vi "XY Plot Commands.vi"(1 "X,Y Log":i32[](array[numeric])=[1, 0], 4 "Plot labels":string[](array[string])=["SR810 cables", "SR810 cables + 1&2", "detector", "cables", "cables + 1&2", "cables + 2&3", "cables + 3&4"], 5 "X,Y Labels":string[](array[string])=["frequency (Hz)", "V\\Brms\\M (V)"], 6 "wavenames":string[](array[string])=["Sum.000003SR810cables", "Sum.000003SR810cables + 1&2", "Sum.000003detector", "Sum.000003cables", "Sum.000003cables+ 1&2", "Sum.000003cables+ 2&3", "Sum.000003cables+ 3&4"]) -> (0 "result string":string="Display 'y_Sum.000003SR810cables' vs 'x_Sum.000003SR810cables'\nAppendToGraph 'y_Sum.000003SR810cables + 1&2' vs 'x_Sum.000003SR810cables + 1&2'\nAppendToGraph 'y_Sum.000003detector' vs 'x_Sum.000003detector'\nAppendToGraph 'y_Sum.000003cables' vs 'x_Sum.000003cables'\nAppendToGraph 'y_Sum.000003cables+ 1&2' vs 'x_Sum.000003cables+ 1&2'\nAppendToGraph 'y_Sum.000003cables+ 2&3' vs 'x_Sum.000003cables+ 2&3'\nAppendToGraph 'y_Sum.000003cables+ 3&4' vs 'x_Sum.000003cables+ 3&4'\nLabel bottom \"frequency (Hz)\"\nLabel left \"V\\Brms\\M (V)\"\nModifyGraph rgb('y_Sum.000003SR810cables')=(65280,0,0)\nModifyGraph rgb('y_Sum.000003SR810cables + 1&2')=(65280,50688,0)\nModifyGraph rgb('y_Sum.000003detector')=(29696,65280,0)\nModifyGraph rgb('y_Sum.000003cables')=(0,65280,20992)\nModifyGraph rgb('y_Sum.000003cables+ 1&2')=(0,60928,65280)\nModifyGraph rgb('y_Sum.000003cables+ 2&3')=(0,10240,65280)\nModifyGraph rgb('y_Sum.000003cables+ 3&4')=(40448,0,65280)\nLegend/C/N=text0/J \"\\\\s('y_Sum.000003SR810cables') SR810 cables\\r\\\\s('y_Sum.000003SR810cables + 1&2') SR810 cables + 1&2\\r\\\\s('y_Sum.000003detector') detector\\r\\\\s('y_Sum.000003cables') cables\\r\\\\s('y_Sum.000003cables+ 1&2') cables + 1&2\\r\\\\s('y_Sum.000003cables+ 2&3') cables + 2&3\\r\\\\s('y_Sum.000003cables+ 3&4') cables + 3&4\"\nModifyGraph mirror=1\nModifyGraph width=216\nModifyGraph height={Aspect,0.6}\n\n\n")   [LabVIEW 2019, in "LV-Data.ITX.lvclass"]
uses:
  LV-Data.ITX.lvclass
  ITX Commands/typedefs/Label--cluster.ctl
  ITX Commands/typedefs/Log--cluster.ctl
  ITX Commands/typedefs/log--enum.ctl
  ITX Commands/ITX Commands.lvclass
panel:
  # "Legend/C/N=text0/J \"\\\\s('y_test.000011Plot9') Plot 9\\r\\\\s('y_test.000011Plot8') Plot 8\""
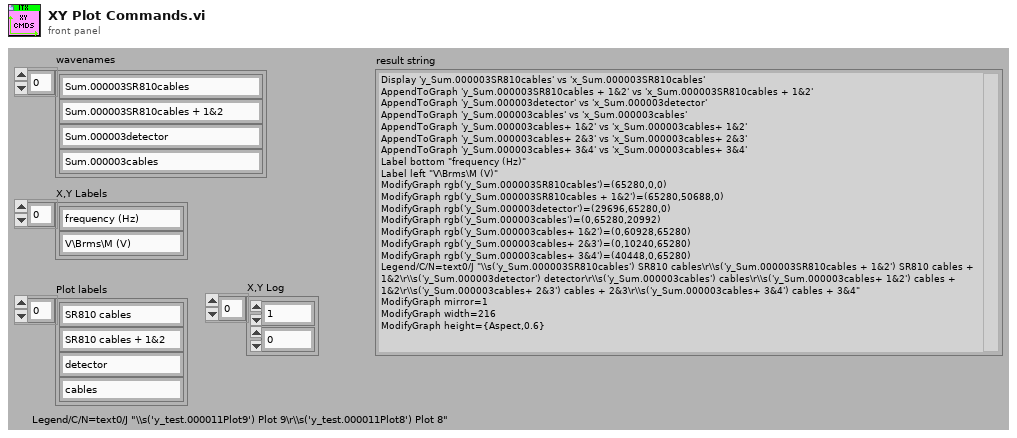
[diagram p1: front panel]
types:
  T1 = typedef "ITX Commands.lvclass/Log--cluster.ctl" = cluster{"bottom":T2, "left":T2}
  T2 = typedef "ITX Commands.lvclass/log--enum.ctl" = enum16{"normal axis", "log base 10", "log base 2"}
  T3 = typedef "ITX Commands.lvclass/Label--cluster.ctl" = cluster{"Bottom":string, "Top":string, "Left":string, "Right":string}
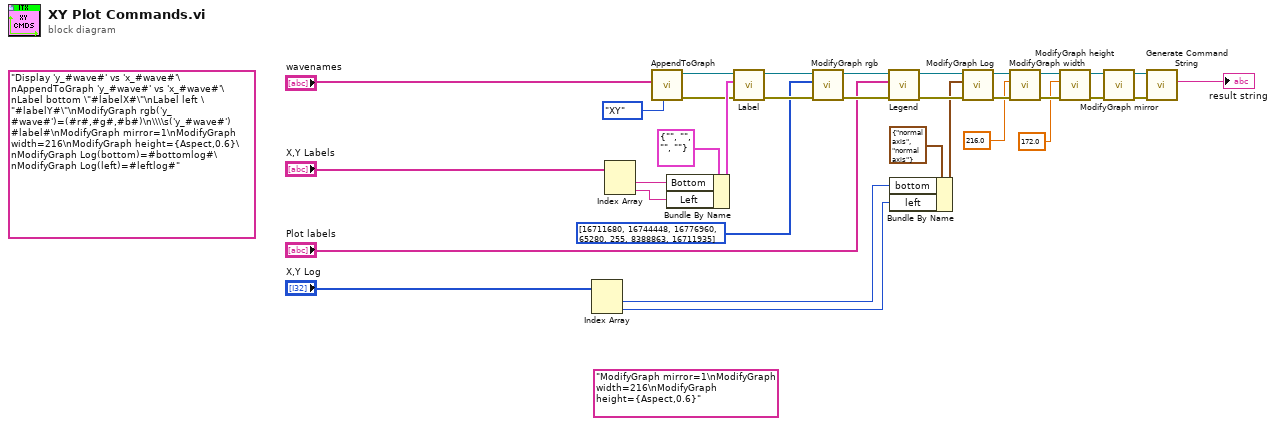
[diagram p0: block diagram]
diagram:
  (unwired) "ModifyGraph mirror=1\nModifyGraph width=216\nModifyGraph height={Aspect,0.6}" ("input string")
  (unwired) "Display 'y_#wave#' vs 'x_#wave#'\nAppendToGraph 'y_#wave#' vs 'x_#wave#'\nLabel bottom \"#labelX#\"\nLabel left \"#labelY#\"\nModifyGraph rgb('y_#wave#')=(#r#,#g#,#b#)\n\\\\s('y_#wave#') #label#\nModifyGraph mirror=1\nModifyGraph width=216\nModifyGraph height={Aspect,0.6}\nModifyGraph Log(bottom)=#bottomlog#\nModifyGraph Log(left)=#leftlog#" ("input string")
  n1 = Index Array(array="X,Y Log") -> (element #1=w18:i32, element #2=w19:i32)  [unwired: 2 in]
  n2 = Index Array(array="X,Y Labels") -> (element #1=w30:string, element #2=w17:string)  [unwired: 2 in]
  n3 = call "AppendToGraph.vi"("Enum"=enum16{"XY", "XY2"}."XY", "wavenames"="wavenames") -> ("error out"=w29:errorcluster, "ITX Commands out"=w31:refnum<class "ITX Commands.lvclass">)  [unwired: 8 in]
  n4 = Bundle By Name(cluster=T3 {"Bottom"="", "Top"="", "Left"="", "Right"=""} ("Label"), "Bottom"=w30, "Left"=w17) -> (w32:T3)
  n5 = call "Label.vi"("error in (no error)"=w29, "Label"=w32, "ITX Commands in"=w31) -> ("error out"=w27:errorcluster, "ITX Commands out"=w28:refnum<class "ITX Commands.lvclass">)  [unwired: 7 in]
  n6 = call "ModifyGraph rgb.vi"("error in (no error)"=w27, "Colorscale"=u32[] [16711680, 16744448, 16776960, 65280, 255, 8388863, 16711935], "ITX Commands in"=w28) -> ("error out"=w26:errorcluster, "ITX Commands out"=w25:refnum<class "ITX Commands.lvclass">)  [unwired: 7 in]
  n7 = call "Legend.vi"("error in (no error)"=w26, "Plot labels"="Plot labels", "ITX Commands in"=w25) -> ("error out"=w23:errorcluster, "ITX Commands out"=w22:refnum<class "ITX Commands.lvclass">)  [unwired: 7 in]
  n8 = Bundle By Name(cluster=T1 {"bottom"=enum."normal axis", "left"=enum."normal axis"} ("Log"), "bottom"=w18, "left"=w19) -> (w20:T1)
  n9 = call "ModifyGraph Log.vi"("error in (no error)"=w23, "Log"=w20, "ITX Commands in"=w22) -> ("error out"=w10:errorcluster, "ITX Commands out"=w9:refnum<class "ITX Commands.lvclass">)  [unwired: 7 in]
  n10 = call "ModifyGraph width.vi"("error in (no error)"=w10, "width (points) [256]"=216.0, "ITX Commands in"=w9) -> ("error out"=w3:errorcluster, "ITX Commands out"=w8:refnum<class "ITX Commands.lvclass">)  [unwired: 7 in]
  n11 = call "ModifyGraph height.vi"("error in (no error)"=w3, "height (points) [256]"=172.0 ("width (points) [256]"), "ITX Commands in"=w8) -> ("error out"=w7:errorcluster, "ITX Commands out"=w6:refnum<class "ITX Commands.lvclass">)  [unwired: 7 in]
  n12 = call "ModifyGraph mirror.vi"("error in (no error)"=w7, "ITX Commands in"=w6) -> ("error out"=w4:errorcluster, "ITX Commands out"=w5:refnum<class "ITX Commands.lvclass">)  [unwired: 8 in]
  n13 = call "Generate Command String.vi"("ITX Commands in"=w5, "error in (no error)"=w4) -> ("ITX Commands"=→"result string":string)  [unwired: 6 in, 2 out]
